vi "UI_Monitor_Data_Setting.vi"() -> ()   [LabVIEW 2014]
panel:
  in  "退出":bool
  in  "保存":bool
  in  "下拉列表":u16(ring) items=["工作条件及报警条件参考值设定", "报警级别设定(开关量)"]
  in  "选项卡控件":enum32{"工作条件及报警条件参考值设定", "报警级别设定(开关量)"}(tab)
  in  "监测参数报警级别":T1 {"性能监测径向位移SRR2" items=["L0", "L1", "L2", "L3"]; "性能监测径向位移SRR1" items=["L0", "L1", "L2", "L3"]; "性能监测径向位移SLR2" items=["L0", "L1", "L2", "L3"]; "性能监测径向位移SLR1" items=["L0", "L1", "L2", "L3"]; "性能监测轴向位移SA" items=["L0", "L1", "L2", "L3"]; "性能监测转速" items=["L0", "L1", "L2", "L3"]; "性能监测轴向油缸力" items=["L0", "L1", "L2", "L3"]; "性能监测径向油缸力" items=["L0", "L1", "L2", "L3"]; "性能监测声发射幅度" items=["L0", "L1", "L2", "L3"]; "性能监测声发射频率" items=["L0", "L1", "L2", "L3"]; "性能监测陪试摩擦力矩" items=["L0", "L1", "L2", "L3"]; "性能监测陪试出油温度" items=["L0", "L1", "L2", "L3"]; "性能监测轴承外圈温度" items=["L0", "L1", "L2", "L3"]; "性能监测外壳振动2" items=["L0", "L1", "L2", "L3"]; "性能监测外壳振动1" items=["L0", "L1", "L2", "L3"]; "性能监测出油温度T2" items=["L0", "L1", "L2", "L3"]; "性能监测出油温度T1" items=["L0", "L1", "L2", "L3"]; "试验油箱1油液温度" items=["L0"]; "试验油箱2油液温度" items=["L0"]; "试验供油压力" items=["L0"]; "陪试供油流量" items=["L0"]; "陪试高压供油压力" items=["L0"]; "陪试低压供油压力" items=["L0"]; "陪试高压供油温度" items=["L0"]; "陪试低压供油温度" items=["L0"]; "齿轮润滑油流量" items=["L0"]; "齿轮润滑油液位" items=["L0"]; "齿轮油箱温度" items=["L0"]; "齿轮冷却装置工作状态" items=["L0"]; "齿轮供油压力" items=["L0"]; "齿轮过滤器压差" items=["L0"]; "齿轮油箱液位" items=["L0"]; "齿轮供油油温" items=["L0"]}
  in  "工作条件及报警条件参考值设定":string[][](table)
  in  "报警信息级别开关量":T2 {"齿轮箱轴承温度异常报警" items=["L0", "L1", "L2", "L3"]; "齿轮箱供油流量过低" items=["L0", "L1", "L2", "L3"]; "陪试单元油箱液位过低" items=["L0", "L1", "L2", "L3"]; "陪试单元油箱液位过高" items=["L0", "L1", "L2", "L3"]; "陪试单元回油过滤器阻塞" items=["L0", "L1", "L2", "L3"]; "陪试单元供油过滤器2阻塞" items=["L0", "L1", "L2", "L3"]; "陪试单元供油过滤器1阻塞" items=["L0", "L1", "L2", "L3"]; "试验单元循环回路过滤器阻塞" items=["L0", "L1", "L2", "L3"]; "试验单元回油过滤器阻塞" items=["L0", "L1", "L2", "L3"]; "试验单元供油过滤器阻塞" items=["L0", "L1", "L2", "L3"]; "试验单元油箱2液位过低" items=["L0", "L1", "L2", "L3"]; "试验单元油箱2液位过高" items=["L0", "L1", "L2", "L3"]; "试验单元油箱1液位过低" items=["L0", "L1", "L2", "L3"]; "试验单元油箱1液位过高" items=["L0", "L1", "L2", "L3"]; "试验单元加热装置异常" items=["L0", "L1", "L2", "L3"]; "加载单元液位过低" items=["L0", "L1", "L2", "L3"]; "加载单元液位过高" items=["L0", "L1", "L2", "L3"]; "加载单元回油过滤器阻塞" items=["L0", "L1", "L2", "L3"]; "加载单元供油过滤器阻塞" items=["L0", "L1", "L2", "L3"]; "齿轮箱油站供油压力过低" items=["L0", "L1", "L2", "L3"]; "齿轮箱油站2号油泵故障" items=["L0", "L1", "L2", "L3"]; "齿轮箱油站1号油泵故障" items=["L0", "L1", "L2", "L3"]; "齿轮箱油站回油过滤器压差过高" items=["L0", "L1", "L2", "L3"]; "齿轮循环回路过滤器压差过高 2" items=["L0", "L1", "L2", "L3"]; "齿轮箱油站供油过滤器压差过高" items=["L0", "L1", "L2", "L3"]; "齿轮箱油站供油油温过高" items=["L0", "L1", "L2", "L3"]; "齿轮箱油站油箱液位过低" items=["L0", "L1", "L2", "L3"]; "齿轮箱油站油箱液位过高" items=["L0", "L1", "L2", "L3"]; "齿轮箱油站冷却装置异常" items=["L0", "L1", "L2", "L3"]; "齿轮箱油站加热装置异常" items=["L0", "L1", "L2", "L3"]; "动力子系统电机转速误差过大" items=["L0", "L1", "L2", "L3"]; "动力子系统电机过载" items=["L0", "L1", "L2", "L3"]; "动力子系统变频器电气参数异常" items=["L0", "L1", "L2", "L3"]; "动力子系统电机温度过高" items=["L0", "L1", "L2", "L3"]}
  in  "报警信息设定（开关量）":string[][](table)
  # "监测参数工作条件及报警条件设置"
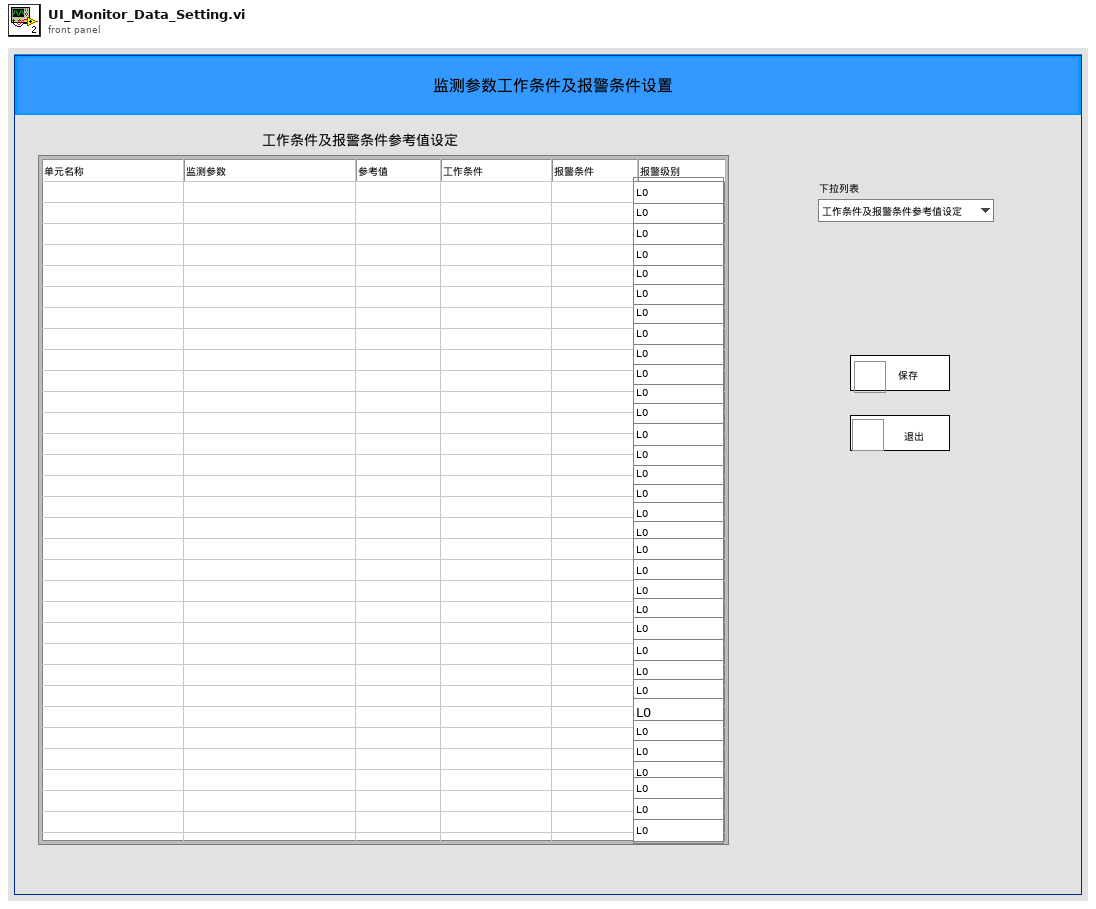
[diagram p1: front panel]
types:
  T1 = cluster{"试验油箱1油液温度":u16, "试验油箱2油液温度":u16, "试验供油压力":u16, "陪试供油流量":u16, "陪试高压供油压力":u16, "陪试低压供油压力":u16, "陪试高压供油温度 ":u16, "陪试低压供油温度":u16, "齿轮润滑油流量":u16, "齿轮润滑油液位":u16, "齿轮油箱温度":u16, "齿轮冷却装置工作状态":u16, "齿轮供油压力":u16, "齿轮过滤器压差":u16, "齿轮油箱液位":u16, "齿轮供油油温":u16, "性能监测出油温度T1":u16, "性能监测出油温度T2":u16, "性能监测外壳振动1":u16, "性能监测外壳振动2":u16, "性能监测轴承外圈温度":u16, "性能监测陪试出油温度":u16, "性能监测陪试摩擦力矩":u16, "性能监测声发射频率":u16, "性能监测声发射幅度":u16, "性能监测径向油缸力":u16, "性能监测轴向油缸力":u16, "性能监测转速":u16, "性能监测轴向位移SA":u16, "性能监测径向位移SLR1":u16, "性能监测径向位移SLR2":u16, "性能监测径向位移SRR1":u16, "性能监测径向位移SRR2":u16}
  T2 = cluster{"加载单元供油过滤器阻塞":u16, "加载单元回油过滤器阻塞":u16, "加载单元液位过高":u16, "加载单元液位过低":u16, "试验单元加热装置异常":u16, "试验单元油箱1液位过高":u16, "试验单元油箱1液位过低":u16, "试验单元油箱2液位过高":u16, "试验单元油箱2液位过低":u16, "试验单元供油过滤器阻塞":u16, "试验单元循环回路过滤器阻塞":u16, "试验单元回油过滤器阻塞":u16, "陪试单元供油过滤器1阻塞":u16, "陪试单元供油过滤器2阻塞":u16, "陪试单元回油过滤器阻塞":u16, "陪试单元油箱液位过高":u16, "陪试单元油箱液位过低":u16, "动力子系统电机温度过高":u16, "动力子系统变频器电气参数异常":u16, "动力子系统电机过载":u16, "动力子系统电机转速误差过大":u16, "齿轮箱油站加热装置异常":u16, "齿轮箱油站冷却装置异常":u16, "齿轮箱油站油箱液位过高":u16, "齿轮箱油站油箱液位过低":u16, "齿轮箱油站供油油温过高":u16, "齿轮箱油站供油过滤器压差过高":u16, "齿轮循环回路过滤器压差过高 2":u16, "齿轮箱油站回油过滤器压差过高":u16, "齿轮箱油站1号油泵故障":u16, "齿轮箱油站2号油泵故障":u16, "齿轮箱油站供油压力过低":u16, "齿轮箱供油流量过低":u16, "齿轮箱轴承温度异常报警":u16}
  T3 = cluster{"[0]":dbl, "[1]":dbl, "[2]":dbl, "[3]":dbl, "[4]":dbl, "[5]":dbl, "[6]":dbl, "[7]":dbl, "[8]":dbl, "[9]":dbl, "[10]":dbl, "[11]":dbl, "[12]":dbl, "[13]":dbl, "[14]":dbl, "[15]":dbl, "[16]":dbl, "[17]":dbl, "[18]":dbl, "[19]":dbl, "[20]":dbl, "[21]":dbl, "[22]":dbl, "[23]":dbl, "[24]":dbl, "[25]":dbl, "[26]":dbl, "[27]":dbl, "[28]":dbl, "[29]":dbl, "[30]":dbl, "[31]":dbl, "[32]":dbl, "[33]":dbl}
  T4 = cluster{"[0]":dbl, "[1]":dbl, "[2]":dbl, "[3]":dbl, "[4]":dbl, "[5]":dbl, "[6]":dbl, "[7]":dbl, "[8]":dbl, "[9]":dbl, "[10]":dbl, "[11]":dbl, "[12]":dbl, "[13]":dbl, "[14]":dbl, "[15]":dbl, "[16]":dbl, "[17]":dbl, "[18]":dbl, "[19]":dbl, "[20]":dbl, "[21]":dbl, "[22]":dbl, "[23]":dbl, "[24]":dbl, "[25]":dbl, "[26]":dbl, "[27]":dbl, "[28]":dbl, "[29]":dbl, "[30]":dbl, "[31]":dbl, "[32]":dbl}
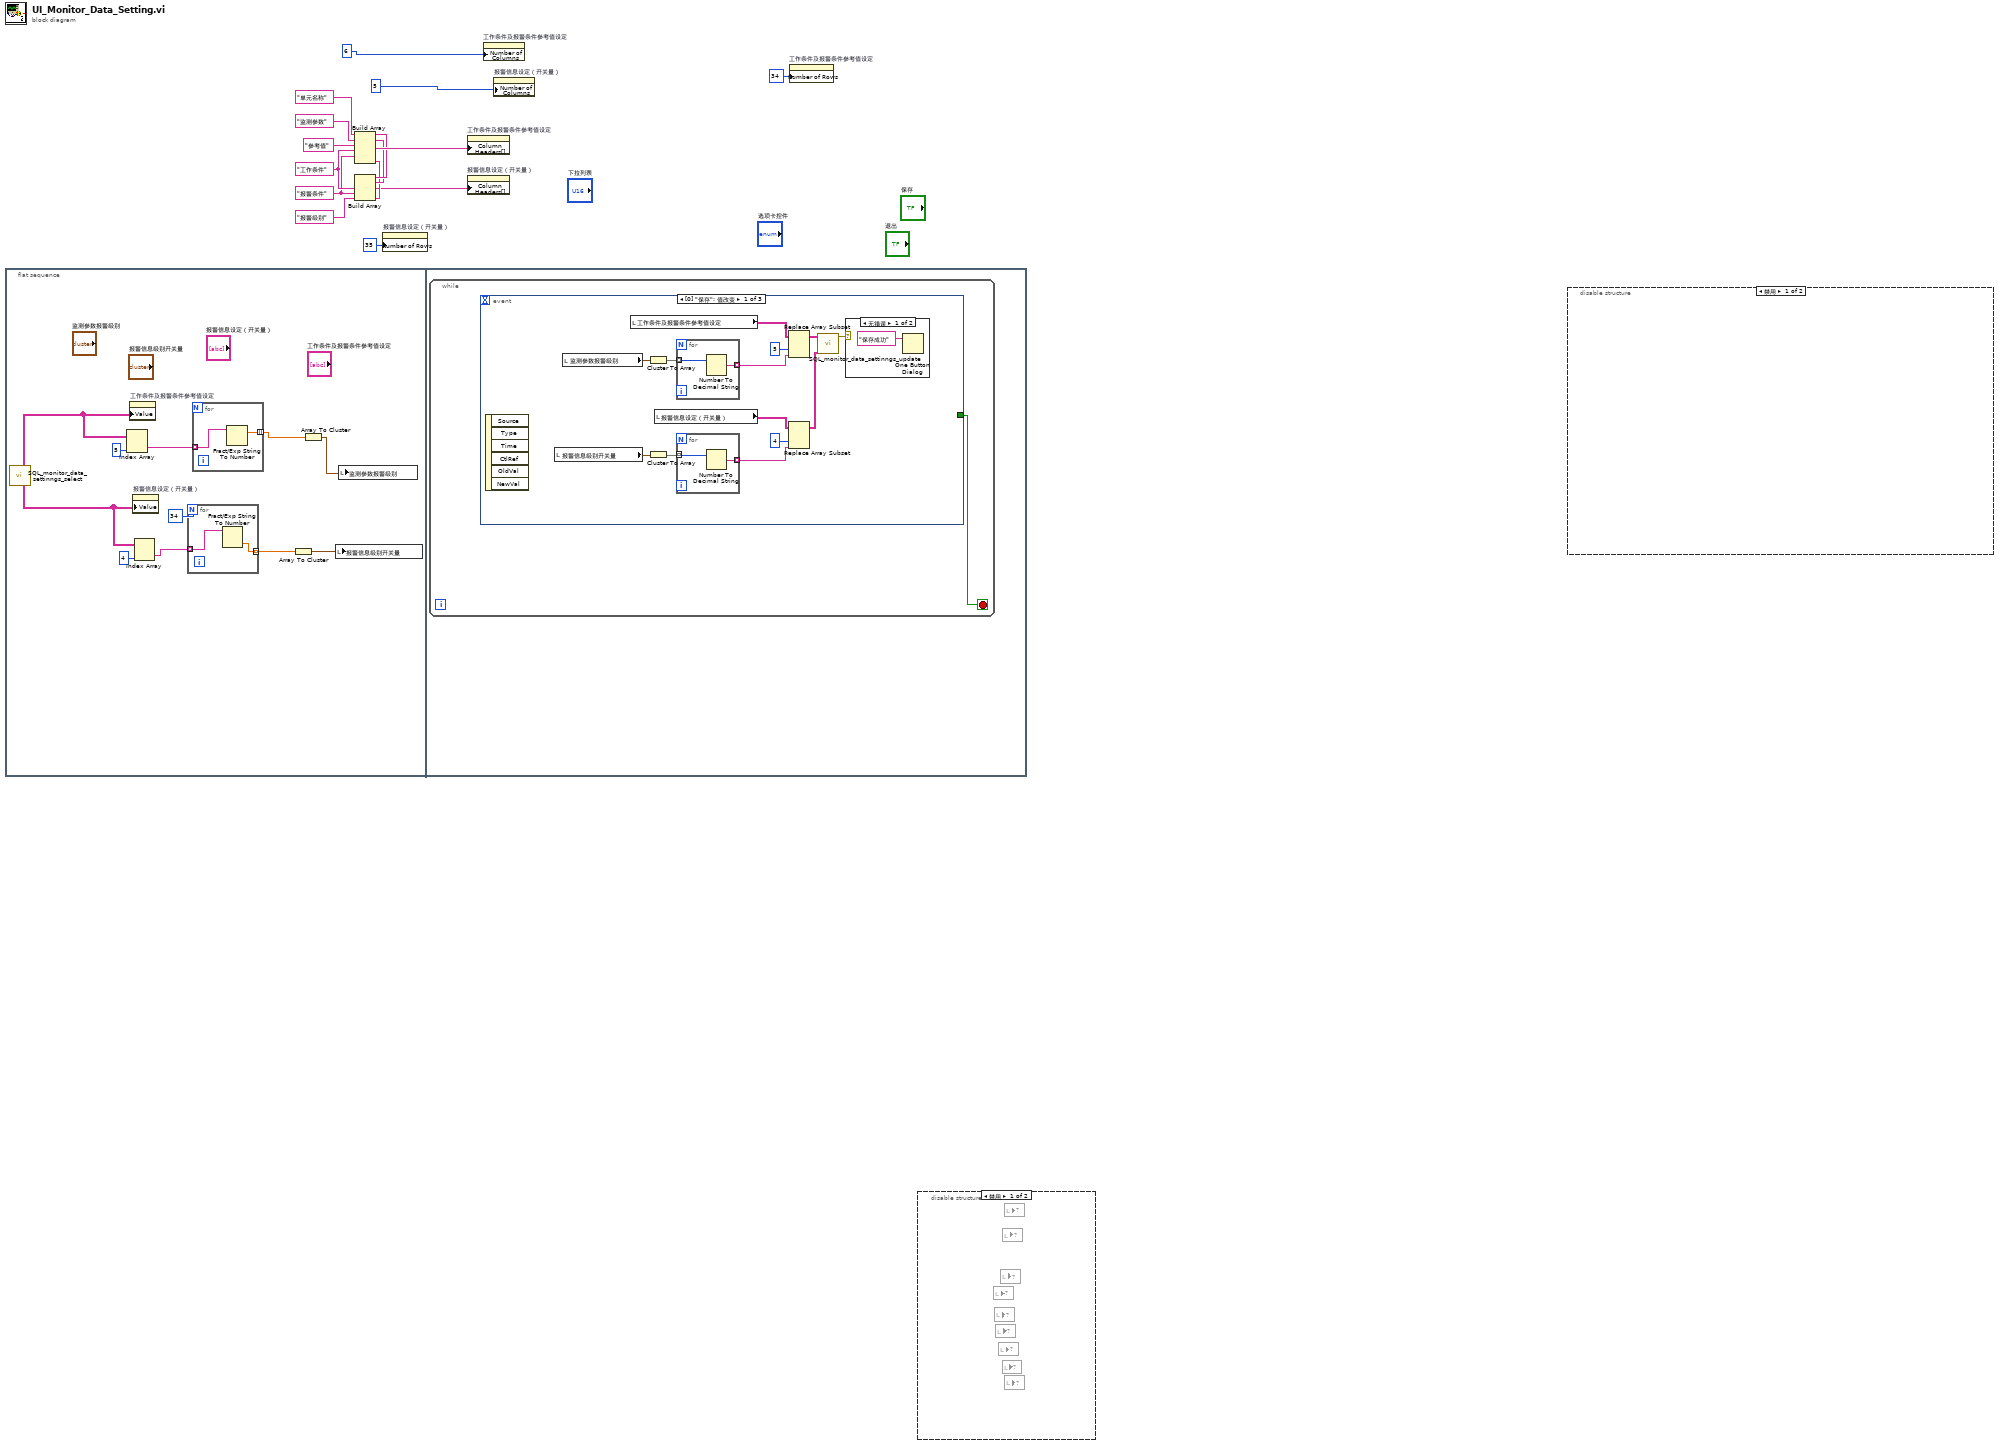
[diagram p0: block diagram]
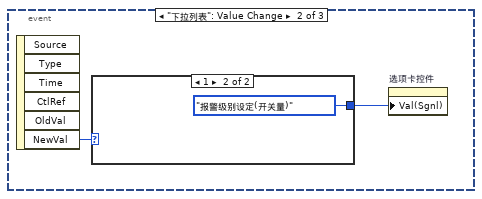
[diagram p5: hidden frame]
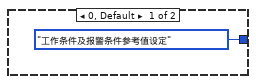
[diagram p6: hidden frame]
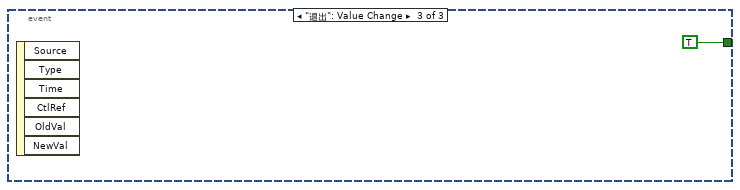
[diagram p7: hidden frame]
diagram:
  w5 = "报警级别"
  w6 = "报警条件"
  w7 = "工作条件"
  w8 = "监测参数"
  w9 = "单元名称"
  n1 = flat-sequence {
    frame #0 {
      n2 = call "SQL_monitor_data_settinngs_select.vi"() -> ("报警级别设置"=w17:string[][], "工作条件及报警门限参考值设定"=w23:string[][])  [unwired: 9 in, 1 out]
      n3 = Index Array(array=w23, index (col)=5 ("禁用的索引 (列)")) -> (element=w21:string[])  [unwired: 1 in]
      n4 = property on="工作条件及报警条件参考值设定" class="Tbl (严格)"("Value"=w23) -> ()  [unwired: 2 in, 2 out]
      n5 = property on="报警信息设定（开关量）" class="Tbl (严格)"("Value"=w17) -> ()  [unwired: 2 in, 2 out]
      n6 = Index Array(array=w17, index (col)=4 ("禁用的索引 (列)")) -> (element=w16:string[])  [unwired: 1 in]
      n7 = for {
        N: 34 -> [_]
        tunnel: w16 -> [w25] mode=indexing
        tunnel: [w24] -> w13 mode=indexing
        n8 = Fract/Exp String To Number(string=w25) -> (number=w24:dbl)  [unwired: 3 in, 1 out]
      }
      n9 = for {
        tunnel: w21 -> [w27] mode=indexing
        tunnel: [w26] -> w20 mode=indexing
        n10 = Fract/Exp String To Number(string=w27) -> (number=w26:dbl)  [unwired: 3 in, 1 out]
      }
      n11 = Array To Cluster(array=w13) -> (cluster=w14:T3)
      n12 = Array To Cluster(array=w20) -> (cluster=w19:T4)
      n13 = local write "报警信息级别开关量"(w14) -> ()
      n14 = local write "监测参数报警级别"(w19) -> ()
    }
    frame #1 {
      n15 = while {
        stop <- w28 stop-if-true
        n16 = event shown="[0] \"保存\": 值改变" {
          selector: _ -> [_ _ _]
          dyn-events: _ -> [_ _ _]
          timeout: _ -> [_ _ _]
          tunnel: [_ _ TRUE] -> w28
          event "保存": Value Change {
            n17 = event-data() -> ()  [unwired: 1 in, 6 out]
            n18 = local read "报警信息级别开关量"() -> (w34:T2)
            n19 = local read "监测参数报警级别"() -> (w39:T1)
            n20 = local read "工作条件及报警条件参考值设定"() -> (w36:string[][])
            n21 = Cluster To Array(cluster=w39) -> (array=w38:u16[])
            n22 = Cluster To Array(cluster=w34) -> (array=w33:u16[])
            n23 = local read "报警信息设定（开关量）"() -> (w32:string[][])
            n24 = for {
              tunnel: w38 -> [w45] mode=indexing
              tunnel: [w44] -> w37 mode=indexing
              n25 = Number To Decimal String(number=w45) -> (decimal integer string=w44:string)  [unwired: 1 in]
            }
            n26 = for {
              tunnel: [w43] -> w31 mode=indexing
              tunnel: w33 -> [w42] mode=indexing
              n27 = Number To Decimal String(number=w42) -> (decimal integer string=w43:string)  [unwired: 1 in]
            }
            n28 = Replace Array Subset(array=w36, new element=w37, index (col)=5 ("禁用的索引 (列)")) -> (w35:string[][])  [unwired: 1 in]
            n29 = Replace Array Subset(array=w32, new element=w31, index (col)=4 ("禁用的索引 (列)")) -> (w29:string[][])  [unwired: 1 in]
            n30 = call "SQL_monitor_data_settinngs_update.vi"("报警信息设置"=w29, "工作条件及报警门限参考值设定"=w35) -> ("error out"=w41:errorcluster)  [unwired: 9 in]
            n31 = case shown="无错误" w41 {
              frame No Error {
                n32 = One Button Dialog(message="保存成功") -> ()  [unwired: 1 in, 1 out]
              }
              frame Error {
              }
            }
          }
          event "下拉列表": Value Change {
            n33 = event-data() -> ("NewVal"=w48:u16)  [unwired: 1 in, 5 out]
            n34 = case shown="1" w48 {
              tunnel: [enum32{"工作条件及报警条件参考值设定", "报警级别设定(开关量)"}."工作条件及报警条件参考值设定" ("值(信号)") enum32{"工作条件及报警条件参考值设定", "报警级别设定(开关量)"}."报警级别设定(开关量)" ("值(信号)")] -> w47
              frame 0, Default {
              }
              frame 1 {
              }
            }
            n35 = property on="选项卡控件" class="TabCtl (严格)"("Val(Sgnl)"=w47) -> ()  [unwired: 2 in, 2 out]
          }
          event "退出": Value Change {
            n36 = event-data() -> ()  [unwired: 1 in, 6 out]
          }
        }
      }
    }
  }
  n37 = Build Array(w9, w8, "参考值", w7, w6, w5) -> (w10:string[])
  n38 = Build Array(w9, w8, w7, w6, w5) -> (w4:string[])
  n39 = property on="报警信息设定（开关量）" class="Tbl (严格)"("Number of Rows"=u32 35 ("行数")) -> ()  [unwired: 2 in, 2 out]
  n40 = property on="工作条件及报警条件参考值设定" class="Tbl (严格)"("Column Headers[]"=w10) -> ()  [unwired: 2 in, 2 out]
  n41 = property on="报警信息设定（开关量）" class="Tbl (严格)"("Column Headers[]"=w4) -> ()  [unwired: 2 in, 2 out]
  n42 = property on="工作条件及报警条件参考值设定" class="Tbl (严格)"("Number of Columns"=6) -> ()  [unwired: 2 in, 2 out]
  n43 = property on="报警信息设定（开关量）" class="Tbl (严格)"("Number of Columns"=5) -> ()  [unwired: 2 in, 2 out]
  n44 = property on="工作条件及报警条件参考值设定" class="Tbl (严格)"("Number of Rows"=u32 34 ("行数")) -> ()  [unwired: 2 in, 2 out]
  n45 = disable-structure shown="禁用" {
    frame Disabled {
      n46 = local read item#-1() -> ()  [unwired: 1 in]
      n47 = local read item#-1() -> ()  [unwired: 1 in]
      n48 = local read item#-1() -> ()  [unwired: 1 in]
      n49 = local read item#-1() -> ()  [unwired: 1 in]
      n50 = local read item#-1() -> ()  [unwired: 1 in]
      n51 = local read item#-1() -> ()  [unwired: 1 in]
      n52 = local read item#-1() -> ()  [unwired: 1 in]
      n53 = local read item#-1() -> ()  [unwired: 1 in]
      n54 = local read item#-1() -> ()  [unwired: 1 in]
    }
    frame Enabled {
    }
  }
  n55 = disable-structure shown="禁用" {
    frame Disabled {
    }
    frame Enabled {
    }
  }
